vi "Close.vi"(0 "Cal Standard Sim in":refnum<class "Cal Standard Sim.lvclass">, 11 "error in (no error)":errorcluster) -> (4 "Cal Standard Sim out":refnum<class "Cal Standard Sim.lvclass">, 15 "error out":errorcluster)   [LabVIEW 2023, in "RFFixtureCharact.Instruments.lvlib" / "Cal Standard Sim.lvclass"]
uses:
  Cal Standard Sim.lvclass
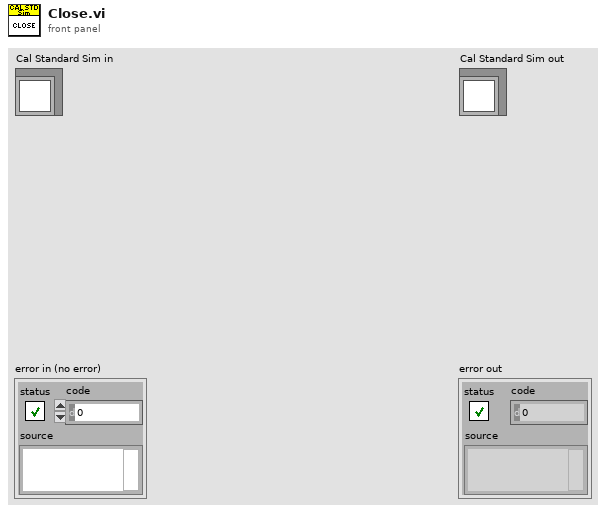
[diagram p1: front panel]
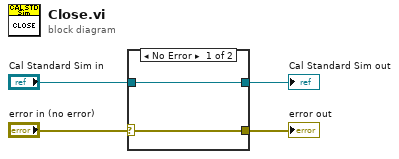
[diagram p0: block diagram]
diagram:
  n1 = case shown="No Error" "error in (no error)" {
    selector: "error in (no error)" -> [w6 w8]
    tunnel: [w6 w8] -> w3
    tunnel: "Cal Standard Sim in" -> [w5 w7]
    tunnel: [w5 w7] -> w1
    frame No Error {
    }
    frame Error {
    }
  }
  "error out" <- w3
  "Cal Standard Sim out" <- w1
